vi "Acquire.vi"(8 "error in (no error)":errorcluster, 9 "Data Queue":refnum<queue>, 10 "Data Notifier":refnum<notifier>, 11 "Hardware Resources in":T1) -> (0 "error out":errorcluster, 3 "Hardware Resources out":T1)   [LabVIEW 2022 SP3, in "Acquisition.lvlib"]
doc: "Perform the acquisition. Replace the contents of this diagram with calls to acquisition hardware."
uses:
  Acquisition.lvlib
  Network Configuration.ctl
  Network JSON.ctl
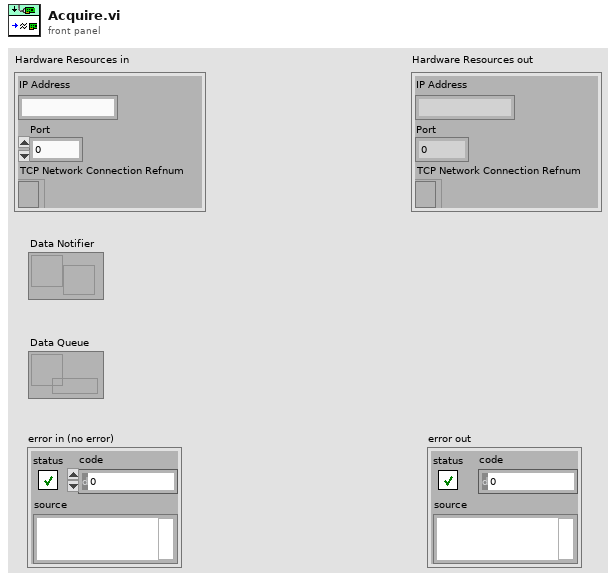
[diagram p1: front panel]
types:
  T1 = typedef "Acquisition.lvlib/Network Configuration.ctl" = cluster{"IP Address":string, "Port":dbl, "TCP Network Connection Refnum":refnum<k5>}
  T2 = cluster{"states":i32[], "timestamp":string, "console":string, "sensors":dbl[]}
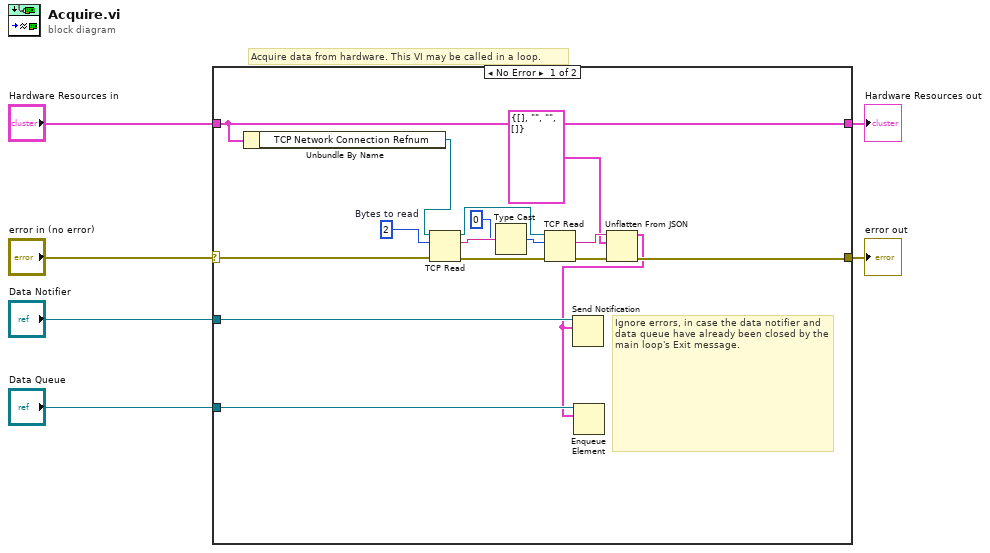
[diagram p0: block diagram]
diagram:
  # "Acquire data from hardware. This VI may be called in a loop."
  n1 = case shown="No Error" "error in (no error)" {
    selector: "error in (no error)" -> [w11 w23]
    tunnel: [w10 w23] -> w5
    tunnel: "Hardware Resources in" -> [w20 w24]
    tunnel: [w20 w24] -> w3
    tunnel: "Data Notifier" -> [w22 _]
    tunnel: "Data Queue" -> [w21 _]
    frame No Error {
      w12 = 2  # Bytes to read
      # "Ignore errors, in case the data notifier and data queue have already been closed by the main loop's Exit message."
      n2 = Unbundle By Name(w20) -> ("TCP Network Connection Refnum"=w7:refnum<k5>)
      n3 = TCP Read(connection ID=w7, bytes to read=w12, error in (no error)=w11) -> (connection ID out=w18:refnum<k5>, data out=w15:string, error out=w13:errorcluster)  [unwired: 2 in]
      n4 = Type Cast(type=u16 0, x=w15) -> (*(type *) &x=w19:u16)
      n5 = TCP Read(connection ID=w18, bytes to read=w19, error in (no error)=w13) -> (data out=w16:string, error out=w17:errorcluster)  [unwired: 2 in, 1 out]
      n6 = Unflatten From JSON(JSON string=w16, type and defaults=T2 {"states"=[], "timestamp"="", "console"="", "sensors"=[]} ("Network JSON"), error in (no error)=w17) -> (value=w8:T2, error out=w10:errorcluster)  [unwired: 4 in]
      n7 = Send Notification(notification=w8, notifier=w22) -> ()  [unwired: 1 in, 2 out]
      n8 = Enqueue Element(queue=w21, element=w8) -> ()  [unwired: 2 in, 3 out]
    }
    frame Error {
    }
  }
  "Hardware Resources out" <- w3
  "error out" <- w5
